vi "Build_Insert_Replace_array.vi"() -> ()   [LabVIEW 2015]
panel:
  out "x-y":dbl
  in  "Enum":enum16{"rep", "Ins", "Buil"}(ring)=enum."Buil"
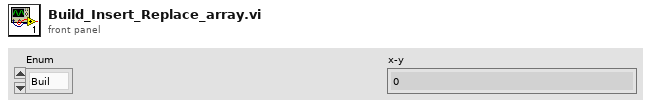
[diagram p1: front panel]
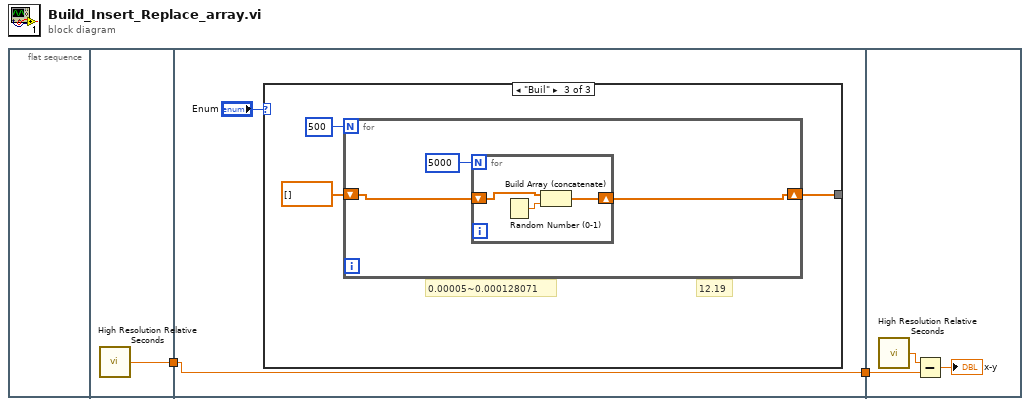
[diagram p0: block diagram]
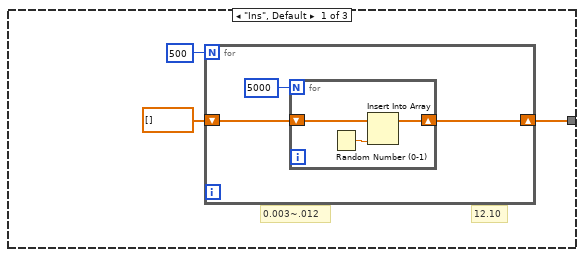
[diagram p2: hidden frame]
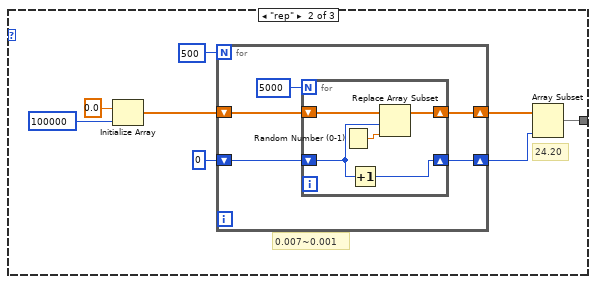
[diagram p3: hidden frame]
diagram:
  n1 = flat-sequence {
    tunnel: [w3] -> w2
    tunnel: w2 -> [w4]
    tunnel: [w4] -> w1
    tunnel: w1 -> [w43]
    frame #0 {
    }
    frame #1 {
      n2 = call <vilib>:"High Resolution Relative Seconds.vi"() -> ("relative seconds"=w3:dbl)
    }
    frame #2 {
      n3 = case shown="\"Buil\"" "Enum" {
        tunnel: [w6 w15 w33] -> _
        frame "Ins", Default {
          # "0.003~.012"
          # "12.10"
          n4 = for {
            N: 500 -> [_]
            shift-right: [w10] -> w6
            shift-left: dbl[] [] ("subarray 2") -> [w11]
            n5 = for {
              N: 5000 -> [_]
              shift-right: [w12] -> w10
              shift-left: w11 -> [w14]
              n6 = Random Number (0-1)() -> (number: 0 to 1=w13:dbl)
              n7 = Insert Into Array(array=w14, new element=w13) -> (w12:dbl[])  [unwired: 1 in]
            }
          }
        }
        frame "rep" {
          # "0.007~0.001"
          # "24.20"
          n8 = Initialize Array(0.0, 100000 ("dimension size")) -> (w21:dbl[])
          n9 = for {
            N: 500 -> [_]
            shift-right: [w27] -> w18
            shift-left: 0 ("dimension size") -> [w24]
            shift-right: [w26] -> w19
            shift-left: w21 -> [w25]
            n10 = for {
              N: 5000 -> [_]
              shift-right: [w31] -> w26
              shift-left: w25 -> [w30]
              shift-right: [w32] -> w27
              shift-left: w24 -> [w28]
              n11 = Random Number (0-1)() -> (number: 0 to 1=w29:dbl)
              n12 = Increment(x=w28) -> (x+1=w32:i32)
              n13 = Replace Array Subset(array=w30, new element=w29, index=w28) -> (w31:dbl[])
            }
          }
          n14 = Array Subset(array=w19, length=w18) -> (w15:dbl[])  [unwired: 1 in]
        }
        frame "Buil" {
          # "0.00005~0.000128071"
          # "12.19"
          n15 = for {
            N: 500 -> [_]
            shift-right: [w37] -> w33
            shift-left: dbl[] [] ("subarray 2") -> [w38]
            n16 = for {
              N: 5000 -> [_]
              shift-right: [w39] -> w37
              shift-left: w38 -> [w41]
              n17 = Random Number (0-1)() -> (number: 0 to 1=w40:dbl)
              n18 = Build Array (concatenate)(w41, w40) -> (w39:dbl[])
            }
          }
        }
      }
    }
    frame #3 {
      n19 = call <vilib>:"High Resolution Relative Seconds.vi"() -> ("relative seconds"=w44:dbl)
      n20 = Subtract(x=w44, y=w43) -> (x-y=→"x-y":dbl)
    }
  }
